vi "UI_Update_Controls.vi"(8 "error in (no error)":errorcluster caption="entrée d'erreur (pas d'erreur)", 9 "ICR Status":T1, 10 "UI Status":T3, 11 "QMH UI References":T2) -> (0 "error out":errorcluster caption="sortie d'erreur", 3 "QMH UI References":T2)   [LabVIEW 2024]
doc: "This VIs updates the controls on the front panel.\nAppearance and values are updated according to the ICR or UI status of the QMH."
uses:
  controls/QMH_UI_References.ctl
  controls/QMH_UI_Command.ctl
  controls/QMH_ICR_Command.ctl
  controls/QMH_UI_Tabs.ctl
  controls/LOOPS_Inputs.ctl
  controls/OPO_Inputs.ctl
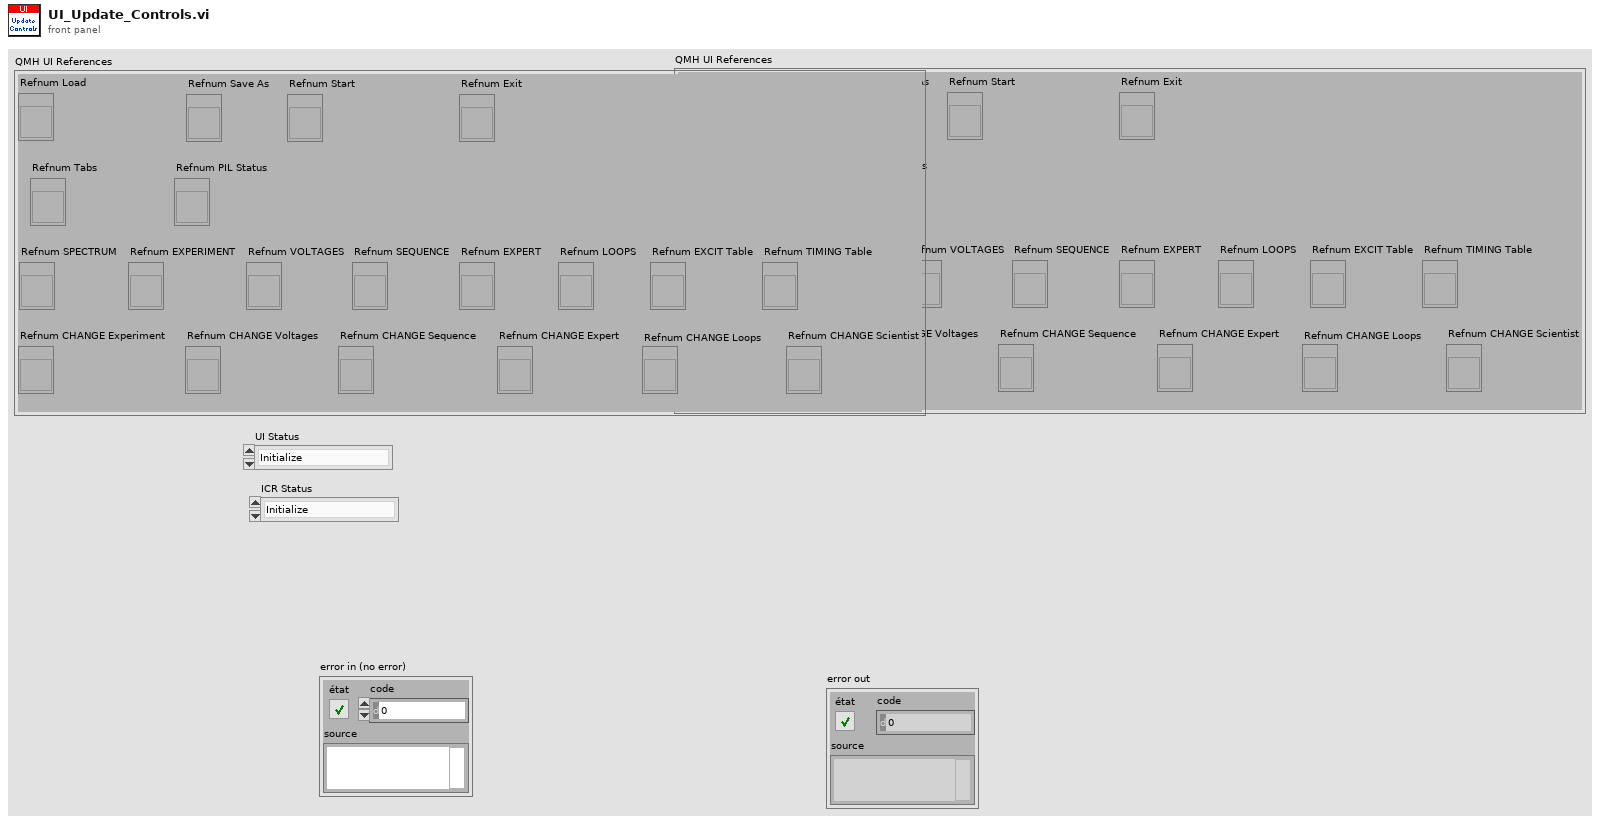
[diagram p1: front panel]
types:
  T1 = typedef "QMH_ICR_Command.ctl" = enum16{"Initialize", "Sequence Loop Setup", "Sequence Setup", "ICR Start", "ICR Stop", "Hardware Setup", "Next Sequence Loop", "Next Accumulation", "Waiting for Trigger", "Sequence Started", "Sequence Finished", "Sequence Loop Done", "Writing Data", "Hardware Reset", "Exit"}
  T2 = typedef "QMH_UI_References.ctl" = cluster{"Refnum Load":refnum<vi>, "Refnum Save As":refnum<vi>, "Refnum Start":refnum<vi>, "Refnum Exit":refnum<vi>, "Refnum Tabs":refnum<vi>, "Refnum SPECTRUM":refnum<vi>, "Refnum EXPERIMENT":refnum<vi>, "Refnum VOLTAGES":refnum<vi>, "Refnum SEQUENCE":refnum<vi>, "Refnum EXPERT":refnum<vi>, "Refnum LOOPS":refnum<vi>, "Refnum EXCIT Table":refnum<vi>, "Refnum TIMING Table":refnum<vi>, "Refnum CHANGE Experiment":refnum<vi>, "Refnum CHANGE Voltages":refnum<vi>, "Refnum CHANGE Sequence":refnum<vi>, "Refnum CHANGE Expert":refnum<vi>, "Refnum CHANGE Loops":refnum<vi>, "Refnum CHANGE Scientist":refnum<vi>, "Refnum PIL Status":refnum<vi>}
  T3 = typedef "QMH_UI_Command.ctl" = enum16{"Initialize", "UI Load", "UI Save", "UI Save As", "UI Change Experiment", "UI Change Voltages", "UI Change Sequence", "UI Change Expert", "UI Change Loops", "UI Change Scientist", "Ready to Start", "UI Start", "Waiting for ICR", "UI Exit", "Update Experiment", "Update Report", "Update ICR Status", "Waiting for User"}
  T4 = typedef "LOOPS_Inputs.ctl" = cluster{"Number of Loops":i16, "Loop Current Value":i16, "OPO Inputs":T5}
  T5 = typedef "OPO_Inputs.ctl" = cluster{"OPO AutoAlignment ON":bool, "OPO Start Value":dbl, "OPO Stop Value":dbl, "OPO Step":dbl}
  T6 = typedef "QMH_UI_Tabs.ctl" = enum32{"Experiment", "Voltages", "Sequence", "Expert", "Loops", "Scientist"}
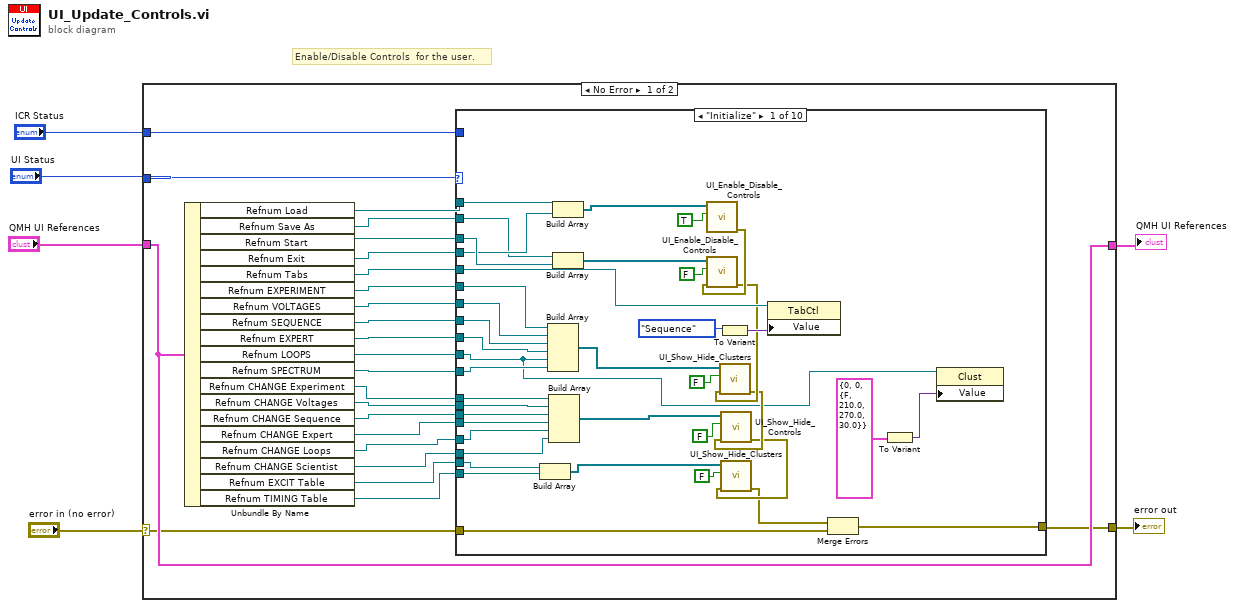
[diagram p0: block diagram]
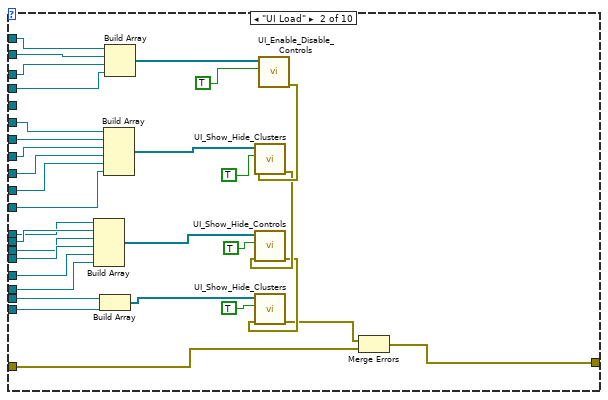
[diagram p2: hidden frame]
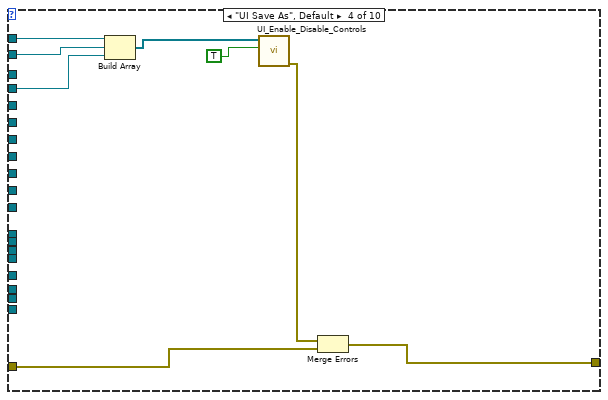
[diagram p4: hidden frame]
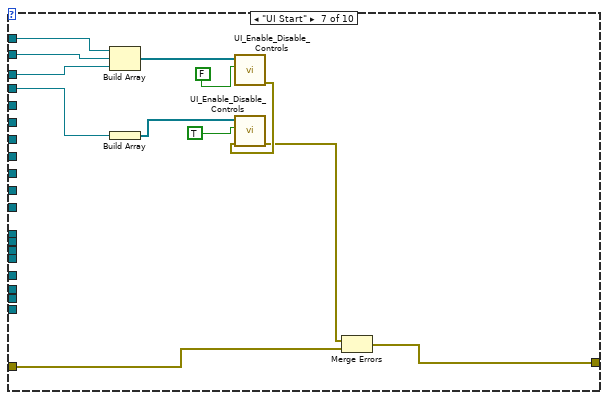
[diagram p7: hidden frame]
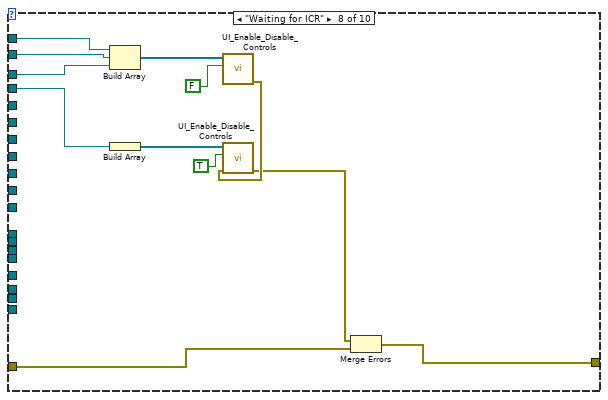
[diagram p8: hidden frame]
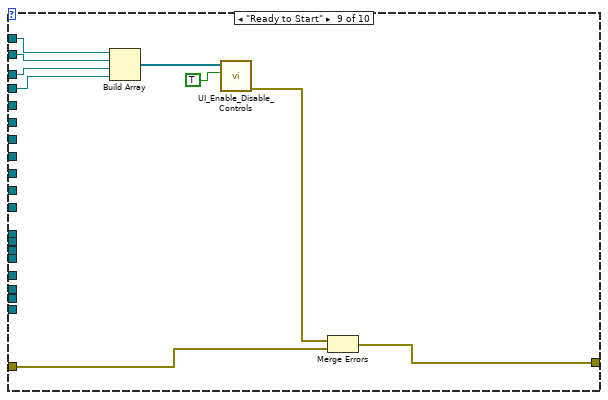
[diagram p9: hidden frame]
diagram:
  # "Enable/Disable Controls  for the user."
  n1 = case shown="No Error" "error in (no error)" {
    selector: "error in (no error)" -> [w15 w149]
    tunnel: [w14 w149] -> w5
    tunnel: "UI Status" -> [w23 _]
    tunnel: "QMH UI References" -> [w17 w148]
    tunnel: [w17 w148] -> w2
    tunnel: "ICR Status" -> [w16 _]
    frame No Error {
      n2 = Unbundle By Name(w17) -> ("Refnum Load"=w30:refnum<vi>, "Refnum Save As"=w18:refnum<vi>, "Refnum Start"=w13:refnum<vi>, "Refnum Exit"=w29:refnum<vi>, "Refnum Tabs"=w28:refnum<vi>, "Refnum EXPERIMENT"=w24:refnum<vi>, "Refnum VOLTAGES"=w25:refnum<vi>, "Refnum SEQUENCE"=w26:refnum<vi>, "Refnum EXPERT"=w27:refnum<vi>, "Refnum LOOPS"=w9:refnum<vi>, "Refnum SPECTRUM"=w8:refnum<vi>, "Refnum CHANGE Experiment"=w22:refnum<vi>, "Refnum CHANGE Voltages"=w21:refnum<vi>, "Refnum CHANGE Sequence"=w20:refnum<vi>, "Refnum CHANGE Expert"=w19:refnum<vi>, "Refnum CHANGE Loops"=w7:refnum<vi>, "Refnum CHANGE Scientist"=w12:refnum<vi>, "Refnum EXCIT Table"=w11:refnum<vi>, "Refnum TIMING Table"=w10:refnum<vi>)
      n3 = case shown="\"Initialize\"" w23 {
        tunnel: w13 -> [w65 w83 _ _ _ _ w119 w131 w142 _]
        tunnel: w30 -> [w68 w100 _ w108 _ _ w118 w130 w144 _]
        tunnel: w29 -> [w64 w84 _ w110 _ _ w123 w135 w141 _]
        tunnel: w28 -> [w62 _ _ _ _ _ _ _ _ _]
        tunnel: w27 -> [w56 w96 _ _ _ _ _ _ _ _]
        tunnel: w26 -> [w57 w95 _ _ _ _ _ _ _ _]
        tunnel: w25 -> [w53 w94 _ _ _ _ _ _ _ _]
        tunnel: w24 -> [w52 w93 _ _ _ _ _ _ _ _]
        tunnel: w22 -> [w51 w87 _ _ _ _ _ _ _ _]
        tunnel: w21 -> [w50 w88 _ _ _ _ _ _ _ _]
        tunnel: w20 -> [w49 w89 _ _ _ _ _ _ _ _]
        tunnel: w19 -> [w48 w90 _ _ _ _ _ _ _ _]
        tunnel: w18 -> [w60 w99 _ w107 _ _ w120 w132 w143 _]
        tunnel: w16 -> [_ _ _ _ _ _ _ _ _ _]
        tunnel: w15 -> [w59 w98 w103 w106 w112 w113 w117 w128 w140 w147]
        tunnel: [w58 w97 w103 w104 w112 w113 w114 w127 w138 w147] -> w14
        tunnel: w12 -> [w31 w73 _ _ _ _ _ _ _ _]
        tunnel: w11 -> [w42 w80 _ _ _ _ _ _ _ _]
        tunnel: w10 -> [w41 w79 _ _ _ _ _ _ _ _]
        tunnel: w9 -> [w35 w74 _ _ _ _ _ _ _ _]
        tunnel: w8 -> [w36 w71 _ _ _ _ _ _ _ _]
        tunnel: w7 -> [w32 w72 _ _ _ _ _ _ _ _]
        frame "Initialize" {
          n4 = Build Array(w42, w41) -> (w40:refnum<vi>[])
          n5 = Build Array(w52, w53, w57, w56, w35, w36) -> (w55:refnum<vi>[])
          n6 = Build Array(w51, w50, w49, w48, w32, w31) -> (w47:refnum<vi>[])
          n7 = Build Array(w68, w64) -> (w67:refnum<vi>[])
          n8 = Build Array(w60, w65) -> (w66:refnum<vi>[])
          n9 = call "UI_Enable_Disable_Controls.vi"("Enable ?"=TRUE ("Activé ?"), "Controls"=w67) -> ("error out"=w45:errorcluster)  [unwired: 9 in]
          n10 = call "UI_Enable_Disable_Controls.vi"("error in (no error)"=w45, "Enable ?"=FALSE ("Activé ?"), "Controls"=w66) -> ("error out"=w44:errorcluster)  [unwired: 8 in]
          n11 = To Variant(anything=QMH_UI_Tabs."Sequence" ("Tabs")) -> (Variant=w63:variant)
          n12 = call "UI_Show_Hide_Clusters.vi"("error in (no error)"=w44, "Enable ?"=FALSE, "Clusters"=w55) -> ("error out"=w43:errorcluster)  [unwired: 8 in]
          n13 = call "UI_Show_Hide_Controls.vi"("error in (no error)"=w43, "Enable ?"=FALSE, "Controls"=w47) -> ("error out"=w38:errorcluster)  [unwired: 8 in]
          n14 = call "UI_Show_Hide_Clusters.vi"("error in (no error)"=w38, "Enable ?"=FALSE, "Clusters"=w40) -> ("error out"=w37:errorcluster)  [unwired: 8 in]
          n15 = property class="TabCtl"(reference=w62, "Value"=w63) -> ()  [unwired: 1 in, 2 out]
          n16 = Merge Errors(w37, w59) -> (w58:errorcluster)
          n17 = To Variant(anything=T4 {"Number of Loops"=0, "Loop Current Value"=0, "OPO Inputs"={"OPO AutoAlignment ON"=FALSE, "OPO Start Value"=210.0, "OPO Stop Value"=270.0, "OPO Step"=30.0}} ("LOOPS Inputs")) -> (Variant=w33:variant)
          n18 = property class="Clust"(reference=w35, "Value"=w33) -> ()  [unwired: 1 in, 2 out]
        }
        frame "UI Load" {
          n19 = Build Array(w87, w88, w89, w90, w72, w73) -> (w86:refnum<vi>[])
          n20 = Build Array(w80, w79) -> (w78:refnum<vi>[])
          n21 = Build Array(w93, w94, w95, w96, w74, w71) -> (w92:refnum<vi>[])
          n22 = Build Array(w100, w99, w83, w84) -> (w101:refnum<vi>[])
          n23 = call "UI_Enable_Disable_Controls.vi"("Enable ?"=TRUE ("Activé ?"), "Controls"=w101) -> ("error out"=w82:errorcluster)  [unwired: 9 in]
          n24 = call "UI_Show_Hide_Clusters.vi"("error in (no error)"=w82, "Enable ?"=TRUE, "Clusters"=w92) -> ("error out"=w81:errorcluster)  [unwired: 8 in]
          n25 = call "UI_Show_Hide_Controls.vi"("error in (no error)"=w81, "Enable ?"=TRUE, "Controls"=w86) -> ("error out"=w76:errorcluster)  [unwired: 8 in]
          n26 = call "UI_Show_Hide_Clusters.vi"("error in (no error)"=w76, "Enable ?"=TRUE, "Clusters"=w78) -> ("error out"=w75:errorcluster)  [unwired: 8 in]
          n27 = Merge Errors(w75, w98) -> (w97:errorcluster)
        }
        frame "UI Save" {
        }
        frame "UI Save As", Default {
          n28 = Build Array(w108, w107, w110) -> (w109:refnum<vi>[])
          n29 = call "UI_Enable_Disable_Controls.vi"("Enable ?"=TRUE ("Activé ?"), "Controls"=w109) -> ("error out"=w105:errorcluster)  [unwired: 9 in]
          n30 = Merge Errors(w105, w106) -> (w104:errorcluster)
        }
        frame "UI Exit" {
        }
        frame "Update Report" {
        }
        frame "UI Start" {
          n31 = Build Array(w118, w120, w119) -> (w121:refnum<vi>[])
          n32 = Build Array(w123) -> (w122:refnum<vi>[])
          n33 = call "UI_Enable_Disable_Controls.vi"("Enable ?"=FALSE ("Activé ?"), "Controls"=w121) -> ("error out"=w116:errorcluster)  [unwired: 9 in]
          n34 = call "UI_Enable_Disable_Controls.vi"("error in (no error)"=w116, "Enable ?"=TRUE ("Activé ?"), "Controls"=w122) -> ("error out"=w115:errorcluster)  [unwired: 8 in]
          n35 = Merge Errors(w115, w117) -> (w114:errorcluster)
        }
        frame "Waiting for ICR" {
          n36 = Build Array(w130, w132, w131) -> (w133:refnum<vi>[])
          n37 = Build Array(w135) -> (w134:refnum<vi>[])
          n38 = call "UI_Enable_Disable_Controls.vi"("Enable ?"=FALSE ("Activé ?"), "Controls"=w133) -> ("error out"=w129:errorcluster)  [unwired: 9 in]
          n39 = call "UI_Enable_Disable_Controls.vi"("error in (no error)"=w129, "Enable ?"=TRUE ("Activé ?"), "Controls"=w134) -> ("error out"=w126:errorcluster)  [unwired: 8 in]
          n40 = Merge Errors(w126, w128) -> (w127:errorcluster)
        }
        frame "Ready to Start" {
          n41 = Build Array(w144, w143, w142, w141) -> (w145:refnum<vi>[])
          n42 = call "UI_Enable_Disable_Controls.vi"("Enable ?"=TRUE ("Activé ?"), "Controls"=w145) -> ("error out"=w139:errorcluster)  [unwired: 9 in]
          n43 = Merge Errors(w139, w140) -> (w138:errorcluster)
        }
        frame "Update ICR Status" {
        }
      }
    }
    frame Error {
    }
  }
  "error out" <- w5
  "QMH UI References" <- w2
